vi "SwerveLatchGoalAngle.vi"(1 "Raw Goal Angle":dbl format="%#_13g", 2 "In Deadband":bool) -> (0 "Latched Goal Angle":dbl)   [LabVIEW 2020]
doc: "Latches the goal azimuth angle when the driver releases the stick. This prevents the modules from slewing to a new orientation and jerking the robot."
uses:
  sensordata.vi
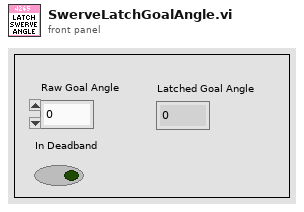
[diagram p1: front panel]
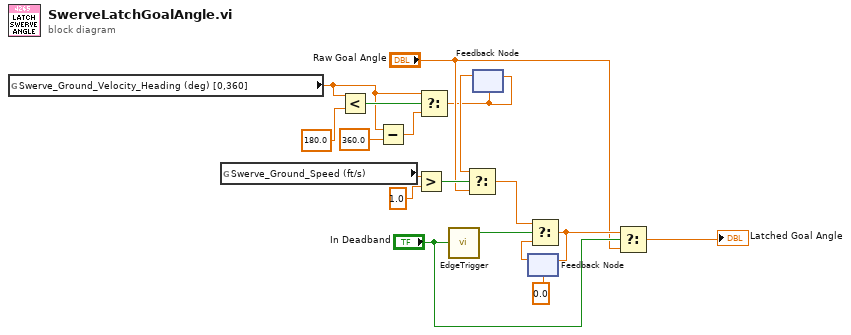
[diagram p0: block diagram]
diagram:
  n1 = global read "sensordata.vi" "Swerve_Ground_Velocity_Heading (deg) [0,360]"() -> (w2:dbl)
  n2 = global read "sensordata.vi" "Swerve_Ground_Speed (ft/s)"() -> (w12:dbl)
  n3 = Less?(x=w2, y=180.0) -> (x < y?=w5:bool)
  n4 = Subtract(x=w2, y=360.0) -> (x-y=w4:dbl)
  n5 = Greater?(x=w12, y=1.0) -> (0:w11:bool)
  n6 = Select(t=w2, s=w5, f=w4) -> (s? t:f=w1:dbl)
  n7 = call "EdgeTrigger.vi"("Input Signal"="In Deadband") -> ("Rising Edge Trigger"=w18:bool)  [unwired: 2 out]
  n8 = feedback-in #1(w1) -> ()
  n9 = feedback #1(w1) -> (w9:dbl)
  n10 = Select(t=w9, s=w11, f="Raw Goal Angle") -> (s? t:f=w7:dbl)
  n11 = feedback #2(0.0) -> (w16:dbl)
  n12 = Select(t=w7, s=w18, f=w16) -> (s? t:f=w15:dbl)
  n13 = feedback-in #2(w15) -> ()
  n14 = Select(t=w15, s="In Deadband", f="Raw Goal Angle") -> (s? t:f=→"Latched Goal Angle":dbl)
